vi "Easy XML Editor Menu.vi"(8 "error in (no error)":errorcluster, 11 "Menu Refnum In":refnum<k9>) -> (0 "error out":errorcluster, 3 "Menu Refnum Out":refnum<k9>)   [LabVIEW 2023]
uses:
  <vilib>/Utility/miscctls.llb/LVMenuShortCut.ctl
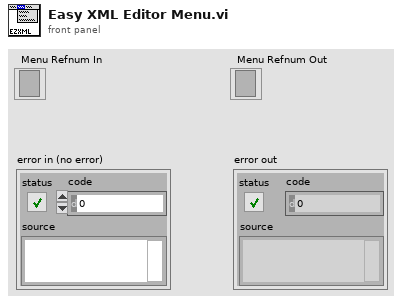
[diagram p1: front panel]
types:
  T1 = typedef "LVMenuShortCut.ctl" = cluster{"Include Shift Key?":bool, "Include Ctrl Key?":bool, "Shortcut Key":string}
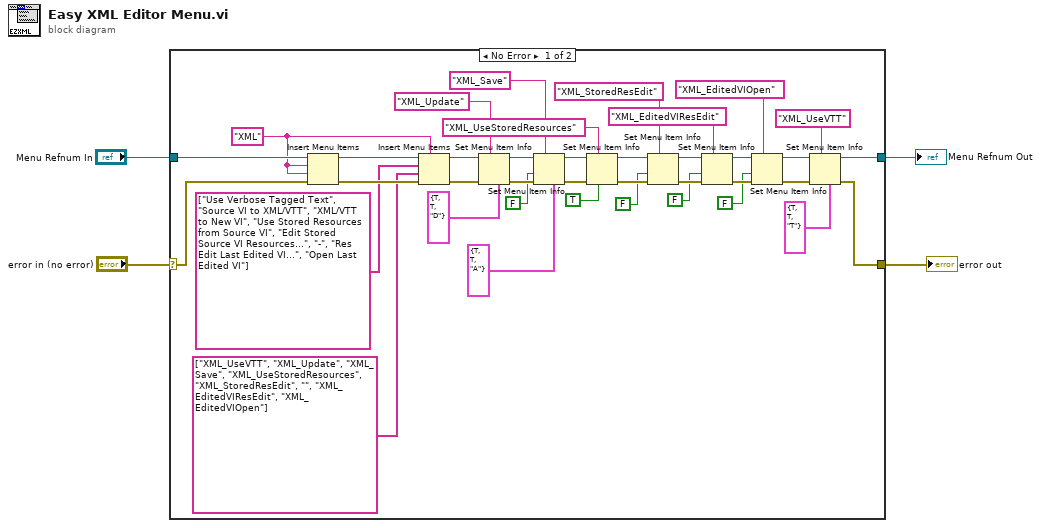
[diagram p0: block diagram]
diagram:
  n1 = case shown="No Error" "error in (no error)" {
    selector: "error in (no error)" -> [w21 w44]
    tunnel: "Menu Refnum In" -> [w42 w43]
    tunnel: [w7 w43] -> w1
    tunnel: [w8 w44] -> w2
    frame No Error {
      w29 = "XML"
      n2 = Insert Menu Items(6:w21, 7:w29, 8:w29, 9:w42) -> (0:w40:errorcluster, 3:w41:refnum<k9>)  [unwired: 2 in, 1 out]
      n3 = Insert Menu Items(5:w29, 6:w40, 7:string[] ["XML_UseVTT", "XML_Update", "XML_Save", "XML_UseStoredResources", "XML_StoredResEdit", "", "XML_EditedVIResEdit", "XML_EditedVIOpen"] ("item tags"), 8:string[] ["Use Verbose Tagged Text", "Source VI to XML/VTT", "XML/VTT to New VI", "Use Stored Resources from Source VI", "Edit Stored Source VI Resources...", "-", "Res Edit Last Edited VI...", "Open Last Edited VI"] ("item names"), 9:w41) -> (0:w36:errorcluster, 3:w37:refnum<k9>)  [unwired: 1 in, 1 out]
      n4 = Set Menu Item Info(4:T1 {"Include Shift Key?"=TRUE, "Include Ctrl Key?"=TRUE, "Shortcut Key"="D"} ("short cut"), 7:"XML_Update", 8:w36, 11:w37) -> (0:w34:errorcluster, 3:w33:refnum<k9>)  [unwired: 3 in]
      n5 = Set Menu Item Info(4:T1 {"Include Shift Key?"=TRUE, "Include Ctrl Key?"=TRUE, "Shortcut Key"="A"} ("short cut"), 7:"XML_Save", 8:w34, 9:FALSE, 11:w33) -> (0:w28:errorcluster, 3:w27:refnum<k9>)  [unwired: 2 in]
      n6 = Set Menu Item Info(6:TRUE, 7:"XML_UseStoredResources" ("item tag"), 8:w28, 11:w27) -> (0:w24:errorcluster, 3:w23:refnum<k9>)  [unwired: 3 in]
      n7 = Set Menu Item Info(7:"XML_StoredResEdit", 8:w24, 9:FALSE, 11:w23) -> (0:w20:errorcluster, 3:w19:refnum<k9>)  [unwired: 3 in]
      n8 = Set Menu Item Info(7:"XML_EditedVIResEdit", 8:w20, 9:FALSE, 11:w19) -> (0:w14:errorcluster, 3:w13:refnum<k9>)  [unwired: 3 in]
      n9 = Set Menu Item Info(7:"XML_EditedVIOpen" ("item tag"), 8:w14, 9:FALSE, 11:w13) -> (0:w9:errorcluster, 3:w10:refnum<k9>)  [unwired: 3 in]
      n10 = Set Menu Item Info(4:T1 {"Include Shift Key?"=TRUE, "Include Ctrl Key?"=TRUE, "Shortcut Key"="T"} ("short cut"), 7:"XML_UseVTT" ("item tag"), 8:w9, 11:w10) -> (0:w8:errorcluster, 3:w7:refnum<k9>)  [unwired: 3 in]
    }
    frame Error {
    }
  }
  "Menu Refnum Out" <- w1
  "error out" <- w2
